vi "LJT4_multi_read.vi"(7 "aNames":string[](array[string]), 8 "error in":errorcluster, 9 "wait_msec":i32=1, 10 "num_read":i32=100, 11 "Handle in":i32) -> (0 "error out":errorcluster, 3 "Handle Out":i32, 4 "status":bool, 5 "data_out":dbl[][](array[numeric]))   [LabVIEW 2019]
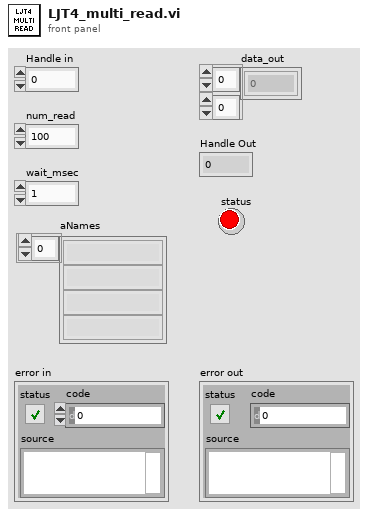
[diagram p1: front panel]
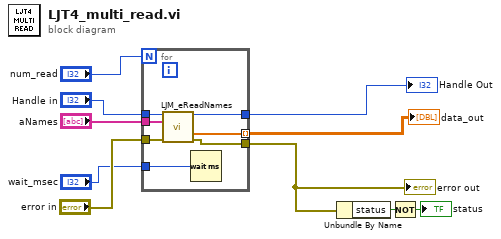
[diagram p0: block diagram]
diagram:
  n1 = for {
    N: "num_read" -> [_]
    tunnel: "Handle in" -> [w17]
    tunnel: "aNames" -> [w16]
    tunnel: "error in" -> [w15]
    tunnel: [w14] -> w4
    tunnel: [w13] -> w3 mode=indexing
    tunnel: [w12] -> w2
    tunnel: "wait_msec" -> [w11]
    n2 = call "LJM_eReadNames.vi"("Handle In"=w17, "aNames"=w16, "error in"=w15) -> ("Handle Out"=w14:i32, "aValuesOut"=w13:dbl[], "error out"=w12:errorcluster)  [unwired: 9 in, 1 out]
    n3 = Wait (ms)(milliseconds to wait=w11) -> ()  [unwired: 1 out]
  }
  "data_out" <- w3
  "error out" <- w2
  "Handle Out" <- w4
  n4 = Unbundle By Name(w2) -> ("status"=w6:bool)
  n5 = Not(x=w6) -> (.not. x?=→"status":bool)
